vi "AverageTestCompile.vi"   [LabVIEW 2013]
uses:
  <vilib>/rvi/Memory/Memory_Emulation/niFpgaMemoryEmulationReadFromVariant.vi
  <vilib>/rvi/Emulation/niFpgaSctlEmulationGetInTimedLoop.vi
  <vilib>/rvi/Memory/Memory_Emulation/niFpgaMemoryEmulationWriteToVariant.vi
  <vilib>/rvi/DataTransferAndStorage/Container/Common/niFpgaContainerGetUniqueNameForEmu.vi
  <vilib>/rvi/FIFO/Fifo_Resource/nirvififoEmulationSetSize.vi
  <vilib>/rvi/Emulation/niFpgaSctlEmulationFifoFullMgr.vi
  <vilib>/rvi/errors/niFpgaSetErrorForExecOnDevCompSimple.vi
  <vilib>/rvi/eio/common/nirviEmuReportErrorAndStop.vi
  <vilib>/rvi/Emulation/niFpgaSctlEmulationResourceMgr.vi
  <vilib>/rvi/Memory/Memory_Emulation/nirvimemoryFastEmulation.vi
  <vilib>/rvi/Memory/Memory_Emulation/nirvimemoryEmulation.vi
  <vilib>/rvi/DataTransferAndStorage/Container/XNode/niFpgaContainer.xnode
  <vilib>/rvi/FIFO/Fifo_Resource/nirvififoEmulationRead.vi
types:
  T1 = cluster{"Accumulated Intensity":u32, "Count":u16}
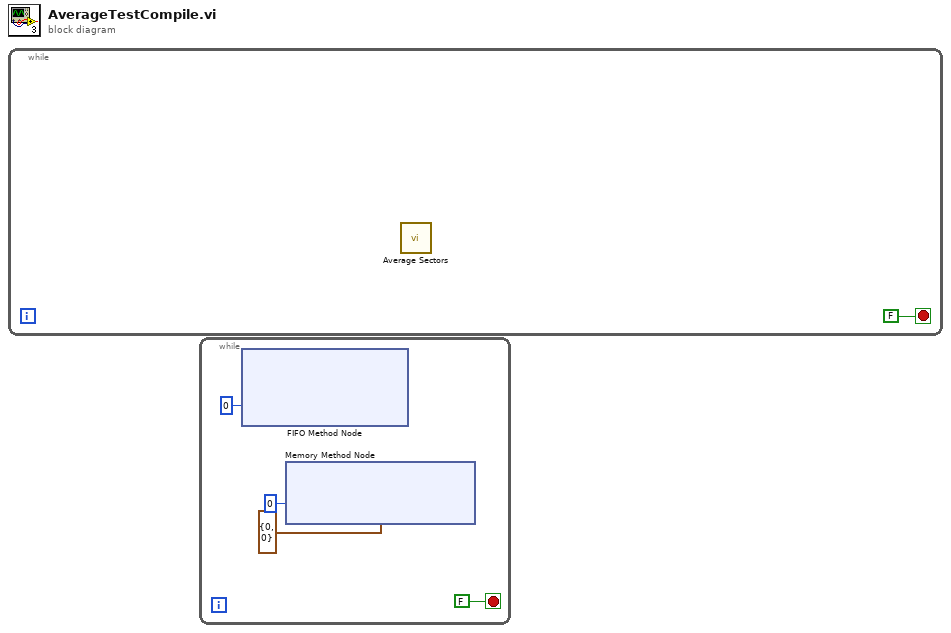
[diagram p0: block diagram]
diagram:
  n1 = while {
    stop <- FALSE stop-if-true
    n2 = call "Average Sectors.vi"() -> ()  [unwired: 12 in]
  }
  n3 = while {
    stop <- FALSE stop-if-true
    n4 = xnode ("FIFO Method Node")("Timeout"=0) -> ()  [unwired: 1 in, 3 out]
    n5 = xnode ("Memory Method Node")("Address"=u32 0, "Data"=T1 {"Accumulated Intensity"=0, "Count"=0}) -> ()  [unwired: 1 in, 1 out]
  }
